vi "wibci filter coefficents.vi"() -> ()   [LabVIEW 2019]
uses:
  <vilib>/addons/Digital Filter Design/Analysis.llb/DFD Plot Freq Response (Linear-Spaced).vi
  <vilib>/addons/Digital Filter Design/NI_DigFilterLicensed.lvlib
panel:
  in  "window":u16(ring) items=["None"=0, "Hanning"=1, "Hamming"=2, "Blackman-Harris"=3, "Exact Blackman"=4, "Blackman"=5, "Flat Top"=6, "4 Term B-Harris"=7, "7 Term B-Harris"=8, "Low Sidelobe"=9, "Triangular"=30, "Kaiser"=60, "Dolph-Chebyshev"=61, "Gaussian"=62]
  out "error out 2":errorcluster
  out "phase response":cluster{"f0":dbl, "df":dbl, "values":dbl[]}[](graph)
  out "magnitude response":cluster{"f0":dbl, "df":dbl, "values":dbl[]}[](graph)
  out "error out":errorcluster
  in  "fs [Hz]":dbl=1.0 format="%.2f"
  in  "low cutoff freq [Hz]":dbl=0.12
  in  "high cutoff freq [Hz]":dbl=0.45
  in  "order":i32=2
  in  "filter type":T1(ring)
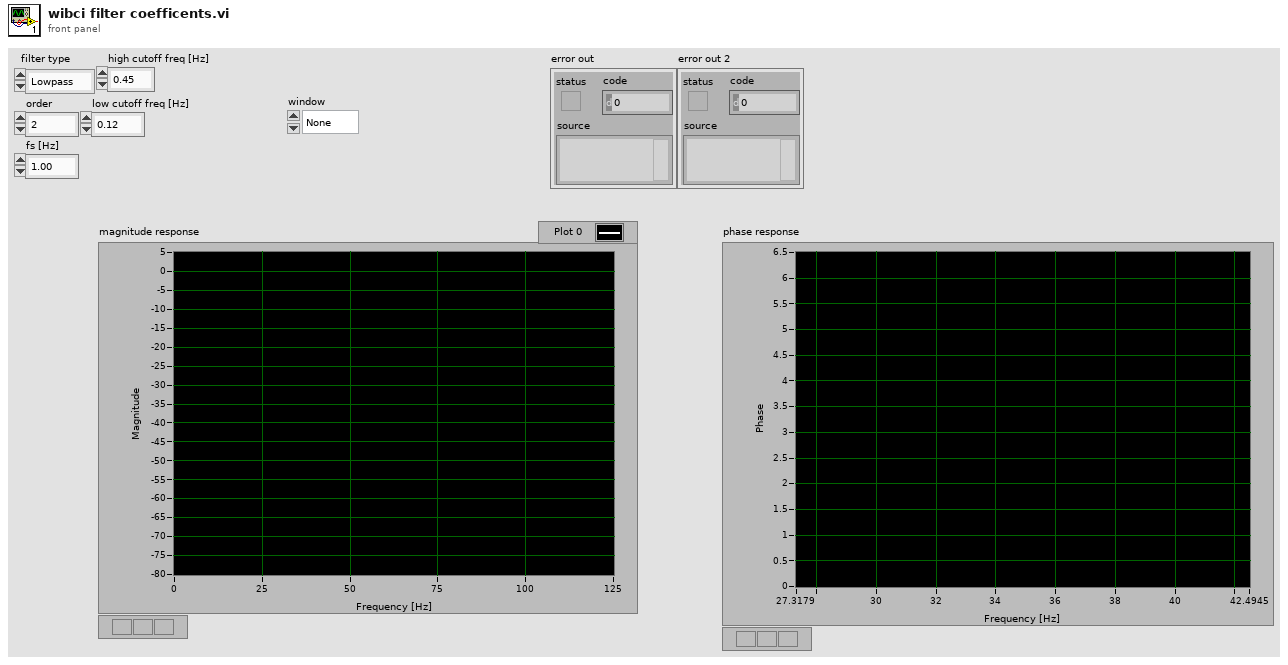
[diagram p1: front panel]
types:
  T1 = enum16{"Lowpass", "Highpass", "Bandpass", "Bandstop"}
  T2 = typedef "NI_DigFilterLicensed.lvlib/DFD Filter Obj.ctl" = cluster{"mSRate_Fs":dbl, "mSRate_Version":string, "mSRate_Comments":string, "mSRate_OrgCoef":T3, "mSRate_CurCoef":T3, "mSRate_Quantized?":bool, "mSRate_QCoef":T3, "mSRate_QSettings":T5[], "mSRate_Order":i32, "mSRate_Scaling":cluster{"mSRate_ScaleByPowerOf2?":bool, "mSRate_ScaleType":T7}}
  T3 = typedef "NI_DigFilterLicensed.lvlib/DFD Filter Coef.ctl" = cluster{"type":T4, "gain":dbl, "coef a (k)":dbl[], "coef b (v)":dbl[]}
  T4 = typedef "NI_DigFilterLicensed.lvlib/DFD Filter Structure Type Selector.ctl" = enum16{"Undefined", "FIR Direct Form", "FIR Direct Form Transposed", "FIR Symmetric", "FIR Antisymmetric", "IIR Direct Form I", "IIR Direct Form I Transposed", "IIR Direct Form II", "IIR Direct Form II Transposed", "IIR Cascaded Second Order Sections Form I", "IIR Cascaded Second Order Sections Form I Transposed", "IIR Cascaded Second Order Sections Form II", "IIR Cascaded Second Order Sections Form II Transposed", "Lattice Allpass (basic sections)", "Lattice Allpass (one multiplier sections)", "Lattice Allpass (normalized sections)", "Lattice AR (basic sections)", "Lattice AR (one multiplier sections)", "Lattice AR (normalized sections)", "Lattice MA (minimum phase)", "Lattice MA (maximum phase)", "Lattice ARMA (basic sections)", "Lattice ARMA (one multiplier sections)", "Lattice ARMA (normalized sections)"}
  T5 = typedef "NI_DigFilterLicensed.lvlib/dfd_Internal Quantization Settings.ctl" = cluster{"source":T6, "wl":i16, "iwl":i16, "overflow mode":enum16{"Saturation", "Wrap"}, "rounding mode":enum16{"Nearest", "Truncation"}, "signed?":bool}
  T6 = typedef "NI_DigFilterLicensed.lvlib/dfd_Internal Quantization Srcs.ctl" = u16
  T7 = typedef "NI_DigFilterLicensed.lvlib/DFD Coef Norm Type.ctl" = enum16{"No Norm", "Time Domain 1-Norm", "Time Domain 2-Norm", "Time Domain Inf-Norm"}
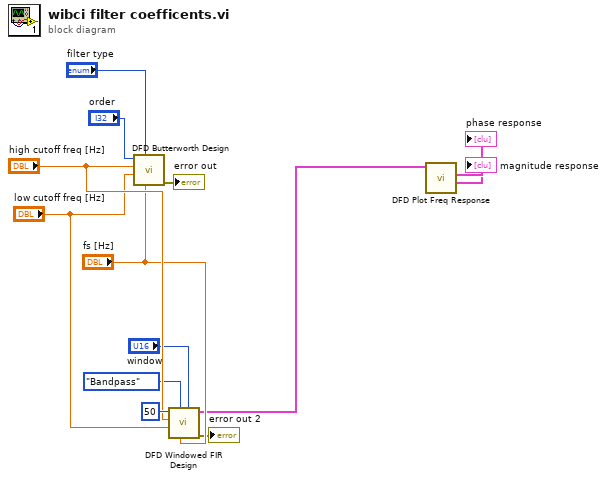
[diagram p0: block diagram]
diagram:
  n1 = call <vilib>:"DFD Butterworth Design.vi"("fs [Hz]"="fs [Hz]", "filter type"="filter type", "low cutoff freq [Hz]"="low cutoff freq [Hz]", "high cutoff freq [Hz]"="high cutoff freq [Hz]", "order"="order") -> ("error out"=→"error out":errorcluster)  [unwired: 5 in, 1 out]
  n2 = call <vilib>:"DFD Windowed FIR Design.vi"("window"="window", "fs [Hz]"="fs [Hz]", "filter type"=T1."Bandpass", "low cutoff freq [Hz]"="low cutoff freq [Hz]", "high cutoff freq [Hz]"="high cutoff freq [Hz]", "order"=50) -> ("error out"=→"error out 2":errorcluster, "filter out"=w1:T2)  [unwired: 4 in]
  n3 = call-poly <vilib>:"DFD Plot Freq Response.vi"("filter in"=w1) -> ("phase response"=→"phase response":cluster{"f0":dbl, "df":dbl, "values":dbl[]}[], "magnitude response"=→"magnitude response":cluster{"f0":dbl, "df":dbl, "values":dbl[]}[])  [unwired: 7 in, 2 out]
